vi "InterruptIRQs.vi"(0 "Occurances":T1) -> ()   [LabVIEW 2019]
uses:
  Controls/Interrupt_Occurances.ctl
  <vilib>/rvi/Emulation/niFpgaGetClockAttributes.vi
  <vilib>/rvi/Emulation/niFpgaSctlEmulationGetInTimedLoop.vi
  <vilib>/rvi/Emulation/niFpgaEmulationReportErrorSimple.vi
  <vilib>/rvi/occurrence/nirviWaitOnOccurrenceBase.vi
  <vilib>/rvi/Emulation/niFpgaCriticalErrorInLSC.vi
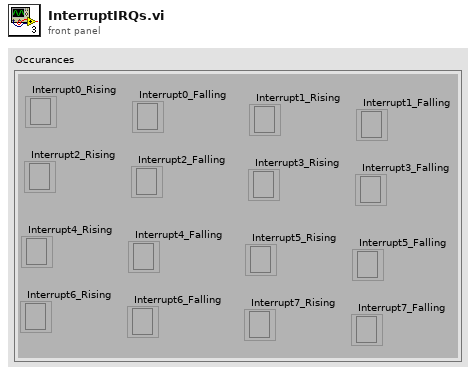
[diagram p1: front panel]
types:
  T1 = typedef "Interrupt_Occurances.ctl" = cluster{"Interrupt0_Rising":refnum<k4>, "Interrupt0_Falling":refnum<k4>, "Interrupt1_Rising":refnum<k4>, "Interrupt1_Falling":refnum<k4>, "Interrupt2_Rising":refnum<k4>, "Interrupt2_Falling":refnum<k4>, "Interrupt3_Rising":refnum<k4>, "Interrupt3_Falling":refnum<k4>, "Interrupt4_Rising":refnum<k4>, "Interrupt4_Falling":refnum<k4>, "Interrupt5_Rising":refnum<k4>, "Interrupt5_Falling":refnum<k4>, "Interrupt6_Rising":refnum<k4>, "Interrupt6_Falling":refnum<k4>, "Interrupt7_Rising":refnum<k4>, "Interrupt7_Falling":refnum<k4>}
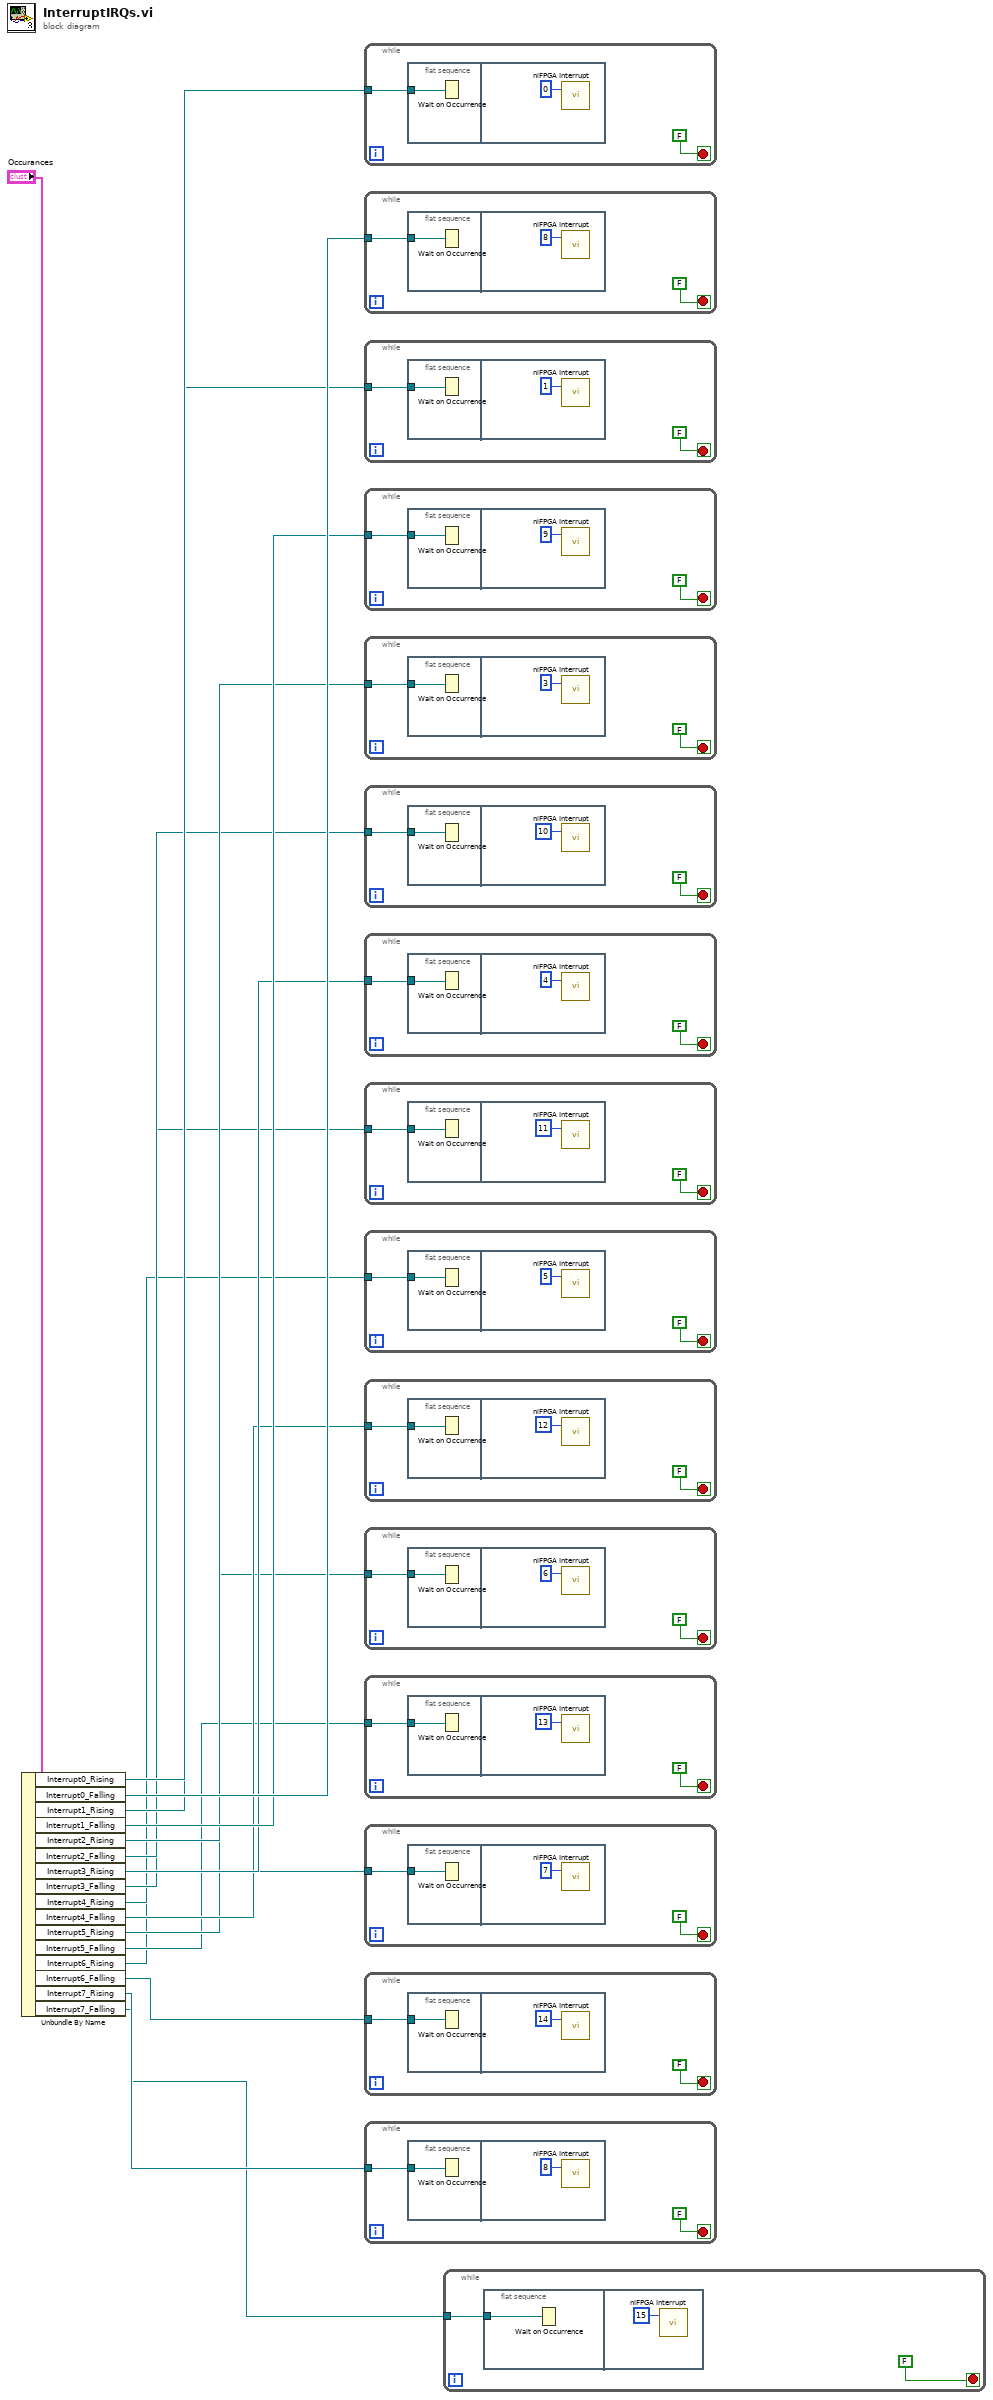
[diagram p0: block diagram]
diagram:
  n1 = Unbundle By Name("Occurances") -> ("Interrupt0_Rising"=w16:refnum<k4>, "Interrupt0_Falling"=w15:refnum<k4>, "Interrupt1_Rising"=w14:refnum<k4>, "Interrupt1_Falling"=w13:refnum<k4>, "Interrupt2_Rising"=w12:refnum<k4>, "Interrupt2_Falling"=w11:refnum<k4>, "Interrupt3_Rising"=w10:refnum<k4>, "Interrupt3_Falling"=w9:refnum<k4>, "Interrupt4_Rising"=w8:refnum<k4>, "Interrupt4_Falling"=w7:refnum<k4>, "Interrupt5_Rising"=w6:refnum<k4>, "Interrupt5_Falling"=w5:refnum<k4>, "Interrupt6_Rising"=w4:refnum<k4>, "Interrupt6_Falling"=w3:refnum<k4>, "Interrupt7_Rising"=w2:refnum<k4>, "Interrupt7_Falling"=w1:refnum<k4>)
  n2 = while {
    tunnel: w16 -> [w18]
    stop <- FALSE stop-if-true
    n3 = flat-sequence {
      tunnel: w18 -> [w20]
      frame #0 {
        n4 = Wait on Occurrence(2:w20) -> ()  [unwired: 2 in, 1 out]
      }
      frame #1 {
        n5 = call <vilib>:"niFPGA Interrupt.vi"("IRQ Number (0)"=u8 0) -> ()  [unwired: 2 in]
      }
    }
  }
  n6 = while {
    tunnel: w15 -> [w22]
    stop <- FALSE stop-if-true
    n7 = flat-sequence {
      tunnel: w22 -> [w24]
      frame #0 {
        n8 = Wait on Occurrence(2:w24) -> ()  [unwired: 2 in, 1 out]
      }
      frame #1 {
        n9 = call <vilib>:"niFPGA Interrupt.vi"("IRQ Number (0)"=u8 8) -> ()  [unwired: 2 in]
      }
    }
  }
  n10 = while {
    tunnel: w14 -> [w26]
    stop <- FALSE stop-if-true
    n11 = flat-sequence {
      tunnel: w26 -> [w28]
      frame #0 {
        n12 = Wait on Occurrence(2:w28) -> ()  [unwired: 2 in, 1 out]
      }
      frame #1 {
        n13 = call <vilib>:"niFPGA Interrupt.vi"("IRQ Number (0)"=u8 1) -> ()  [unwired: 2 in]
      }
    }
  }
  n14 = while {
    tunnel: w13 -> [w30]
    stop <- FALSE stop-if-true
    n15 = flat-sequence {
      tunnel: w30 -> [w32]
      frame #0 {
        n16 = Wait on Occurrence(2:w32) -> ()  [unwired: 2 in, 1 out]
      }
      frame #1 {
        n17 = call <vilib>:"niFPGA Interrupt.vi"("IRQ Number (0)"=u8 9) -> ()  [unwired: 2 in]
      }
    }
  }
  n18 = while {
    tunnel: w12 -> [w34]
    stop <- FALSE stop-if-true
    n19 = flat-sequence {
      tunnel: w34 -> [w36]
      frame #0 {
        n20 = Wait on Occurrence(2:w36) -> ()  [unwired: 2 in, 1 out]
      }
      frame #1 {
        n21 = call <vilib>:"niFPGA Interrupt.vi"("IRQ Number (0)"=u8 3) -> ()  [unwired: 2 in]
      }
    }
  }
  n22 = while {
    tunnel: w11 -> [w38]
    stop <- FALSE stop-if-true
    n23 = flat-sequence {
      tunnel: w38 -> [w40]
      frame #0 {
        n24 = Wait on Occurrence(2:w40) -> ()  [unwired: 2 in, 1 out]
      }
      frame #1 {
        n25 = call <vilib>:"niFPGA Interrupt.vi"("IRQ Number (0)"=u8 10) -> ()  [unwired: 2 in]
      }
    }
  }
  n26 = while {
    tunnel: w10 -> [w42]
    stop <- FALSE stop-if-true
    n27 = flat-sequence {
      tunnel: w42 -> [w44]
      frame #0 {
        n28 = Wait on Occurrence(2:w44) -> ()  [unwired: 2 in, 1 out]
      }
      frame #1 {
        n29 = call <vilib>:"niFPGA Interrupt.vi"("IRQ Number (0)"=u8 4) -> ()  [unwired: 2 in]
      }
    }
  }
  n30 = while {
    tunnel: w9 -> [w46]
    stop <- FALSE stop-if-true
    n31 = flat-sequence {
      tunnel: w46 -> [w48]
      frame #0 {
        n32 = Wait on Occurrence(2:w48) -> ()  [unwired: 2 in, 1 out]
      }
      frame #1 {
        n33 = call <vilib>:"niFPGA Interrupt.vi"("IRQ Number (0)"=u8 11) -> ()  [unwired: 2 in]
      }
    }
  }
  n34 = while {
    tunnel: w8 -> [w50]
    stop <- FALSE stop-if-true
    n35 = flat-sequence {
      tunnel: w50 -> [w52]
      frame #0 {
        n36 = Wait on Occurrence(2:w52) -> ()  [unwired: 2 in, 1 out]
      }
      frame #1 {
        n37 = call <vilib>:"niFPGA Interrupt.vi"("IRQ Number (0)"=u8 5) -> ()  [unwired: 2 in]
      }
    }
  }
  n38 = while {
    tunnel: w7 -> [w54]
    stop <- FALSE stop-if-true
    n39 = flat-sequence {
      tunnel: w54 -> [w56]
      frame #0 {
        n40 = Wait on Occurrence(2:w56) -> ()  [unwired: 2 in, 1 out]
      }
      frame #1 {
        n41 = call <vilib>:"niFPGA Interrupt.vi"("IRQ Number (0)"=u8 12) -> ()  [unwired: 2 in]
      }
    }
  }
  n42 = while {
    tunnel: w6 -> [w58]
    stop <- FALSE stop-if-true
    n43 = flat-sequence {
      tunnel: w58 -> [w60]
      frame #0 {
        n44 = Wait on Occurrence(2:w60) -> ()  [unwired: 2 in, 1 out]
      }
      frame #1 {
        n45 = call <vilib>:"niFPGA Interrupt.vi"("IRQ Number (0)"=u8 6) -> ()  [unwired: 2 in]
      }
    }
  }
  n46 = while {
    tunnel: w5 -> [w62]
    stop <- FALSE stop-if-true
    n47 = flat-sequence {
      tunnel: w62 -> [w64]
      frame #0 {
        n48 = Wait on Occurrence(2:w64) -> ()  [unwired: 2 in, 1 out]
      }
      frame #1 {
        n49 = call <vilib>:"niFPGA Interrupt.vi"("IRQ Number (0)"=u8 13) -> ()  [unwired: 2 in]
      }
    }
  }
  n50 = while {
    tunnel: w4 -> [w66]
    stop <- FALSE stop-if-true
    n51 = flat-sequence {
      tunnel: w66 -> [w68]
      frame #0 {
        n52 = Wait on Occurrence(2:w68) -> ()  [unwired: 2 in, 1 out]
      }
      frame #1 {
        n53 = call <vilib>:"niFPGA Interrupt.vi"("IRQ Number (0)"=u8 7) -> ()  [unwired: 2 in]
      }
    }
  }
  n54 = while {
    tunnel: w3 -> [w70]
    stop <- FALSE stop-if-true
    n55 = flat-sequence {
      tunnel: w70 -> [w72]
      frame #0 {
        n56 = Wait on Occurrence(2:w72) -> ()  [unwired: 2 in, 1 out]
      }
      frame #1 {
        n57 = call <vilib>:"niFPGA Interrupt.vi"("IRQ Number (0)"=u8 14) -> ()  [unwired: 2 in]
      }
    }
  }
  n58 = while {
    tunnel: w2 -> [w74]
    stop <- FALSE stop-if-true
    n59 = flat-sequence {
      tunnel: w74 -> [w76]
      frame #0 {
        n60 = Wait on Occurrence(2:w76) -> ()  [unwired: 2 in, 1 out]
      }
      frame #1 {
        n61 = call <vilib>:"niFPGA Interrupt.vi"("IRQ Number (0)"=u8 8) -> ()  [unwired: 2 in]
      }
    }
  }
  n62 = while {
    tunnel: w1 -> [w78]
    stop <- FALSE stop-if-true
    n63 = flat-sequence {
      tunnel: w78 -> [w80]
      frame #0 {
        n64 = Wait on Occurrence(2:w80) -> ()  [unwired: 2 in, 1 out]
      }
      frame #1 {
        n65 = call <vilib>:"niFPGA Interrupt.vi"("IRQ Number (0)"=u8 15) -> ()  [unwired: 2 in]
      }
    }
  }
